vi "Read Reset With Defaults.vi"(8 "error in (no error)":errorcluster, 11 "CS++DeviceActor in":refnum<class "CS++DeviceActor.lvclass">) -> (0 "error out":errorcluster, 2 "Reset With Defaults":bool, 3 "CS++DeviceActor out":refnum<class "CS++DeviceActor.lvclass">)   [LabVIEW 2016, in "CS++DeviceActor.lvlib" / "CS++DeviceActor.lvclass"]
doc: "Read option Reset With Defaults."
uses:
  CS++DeviceActor.lvclass
  CS++DeviceActor.lvclass/CS++DeviceActor.ctl
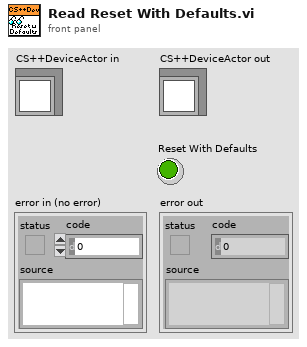
[diagram p1: front panel]
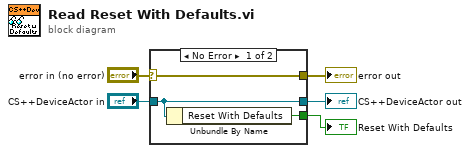
[diagram p0: block diagram]
diagram:
  n1 = case shown="No Error" "error in (no error)" {
    selector: "error in (no error)" -> [w8 w9]
    tunnel: [w8 w9] -> w4
    tunnel: [w7 w10] -> w2
    tunnel: "CS++DeviceActor in" -> [w7 w10]
    tunnel: [w6 _] -> w1
    frame No Error {
      n2 = Unbundle By Name(w7) -> ("Reset With Defaults"=w6:bool)
    }
    frame Error {
    }
  }
  "error out" <- w4
  "CS++DeviceActor out" <- w2
  "Reset With Defaults" <- w1
